vi "Reset_timer.vi"() -> ()   [LabVIEW 2020]
doc: "Przechowuje informację czy należy zresetować timer."
panel:
  out "Boolean":bool
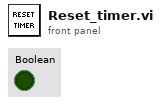
[diagram p1: front panel]
diagram:
